vi "Log UI Cmd.vi"(8 "error in (no error)":errorcluster, 10 "UI Process Command in":refnum<class "Generic UI Process Command.lvclass">, 11 "UI Process Data in":T1) -> (0 "error out":errorcluster, 3 "UI Process Data out":T1)   [LabVIEW 2019, in "User Interface Process.lvlib" / "Generic UI Process Command.lvclass"]
uses:
  Generic UI Process Command.lvclass
  UI Process Data.ctl
  TS Framework/ExeLogging/UI Logger/UI Logger.lvclass
  UI State.ctl
  Generic UI Process Command.lvclass/Generic UI Process Command.ctl
  User Interface Process.lvlib
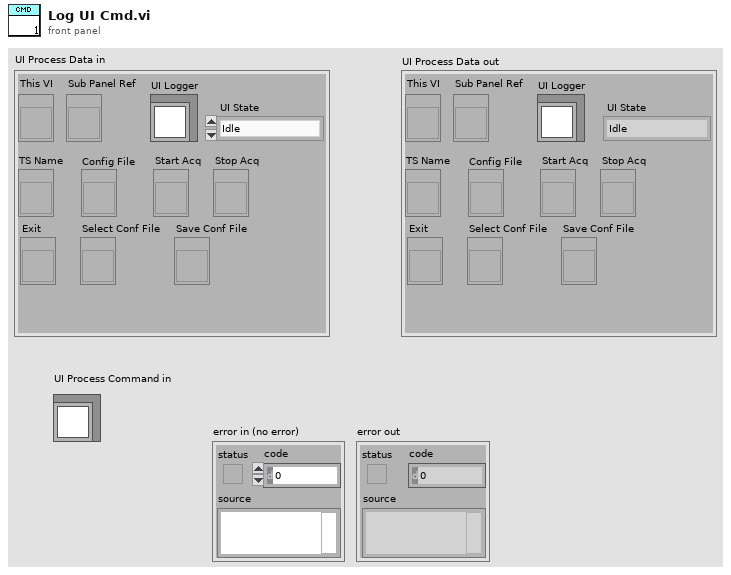
[diagram p1: front panel]
types:
  T1 = typedef "User Interface Process.lvlib/UI Process Data.ctl" = cluster{"This VI":refnum<vi>, "Sub Panel Ref":refnum<vi>, "UI Logger":refnum<class "UI Logger.lvclass">, "TS Name":refnum<vi>, "Config File":refnum<vi>, "Start Acq":refnum<vi>, "Stop Acq":refnum<vi>, "Exit":refnum<vi>, "Select Conf File":refnum<vi>, "Save Conf File":refnum<vi>, "UI State":T2}
  T2 = typedef "User Interface Process.lvlib/UI State.ctl" = enum16{"Idle", "Acquiring"}
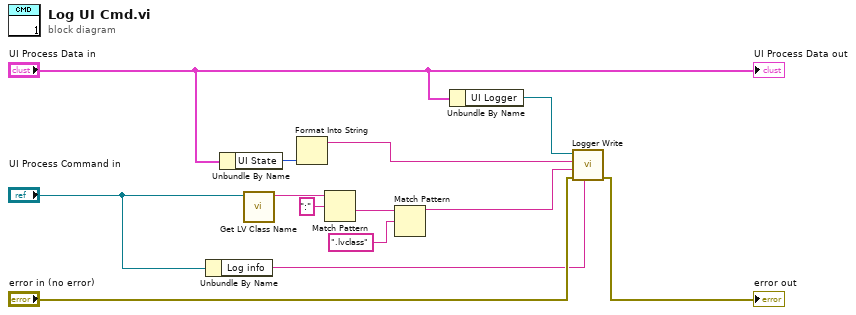
[diagram p0: block diagram]
diagram:
  n1 = Unbundle By Name("UI Process Command in") -> ("Log info"=w8:string)
  n2 = Unbundle By Name("UI Process Data in") -> ("UI State"=w7:T2)
  n3 = call <vilib>:"Get LV Class Name.vi"("object"="UI Process Command in") -> ("class name"=w10:string)  [unwired: 9 in, 1 out]
  n4 = Format Into String(w7) -> (resulting string=w6:string)  [unwired: 3 in, 1 out]
  n5 = Match Pattern(string=w10, regular expression=":") -> (after substring=w5:string)  [unwired: 1 in, 3 out]
  n6 = Match Pattern(string=w5, regular expression=".lvclass") -> (before substring=w3:string)  [unwired: 1 in, 3 out]
  n7 = Unbundle By Name("UI Process Data in") -> ("UI Logger"=w11:refnum<class "UI Logger.lvclass">)
  n8 = call-dynamic "Logger Write.vi"("Extra"=w8, "error in (no error)"="error in (no error)", "Command"=w3, "State"=w6, "Logger in"=w11) -> ("error out"=→"error out":errorcluster)  [unwired: 6 in]
  "UI Process Data out" <- "UI Process Data in"
